vi "Launch.vi"(6 "Only Init (F)":bool, 7 "API Type (Base)":refnum<class "Actor API.lvclass">, 8 "error in (no error)":errorcluster, 11 "Actor in":refnum<class "Actor.lvclass">) -> (0 "error out":errorcluster, 3 "Actor API":refnum<class "Actor API.lvclass">)   [LabVIEW 2022 SP3, in "Artifex.lvlib" / "Actor.lvclass"]
uses:
  Actor.lvclass
  Priority Message Queue/Priority Message Queue.lvclass
  Actor Proxy/Actor API.lvclass
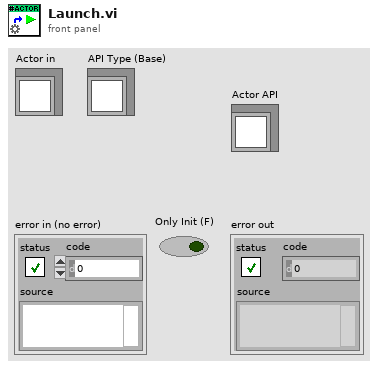
[diagram p1: front panel]
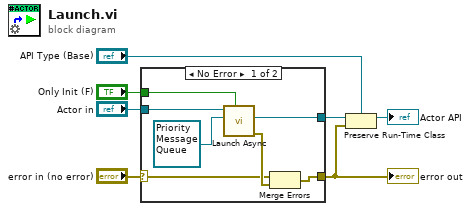
[diagram p0: block diagram]
diagram:
  n1 = case shown="No Error" "error in (no error)" {
    selector: "error in (no error)" -> [w13 w15]
    tunnel: "Actor in" -> [w8 _]
    tunnel: [w12 w15] -> w4
    tunnel: [w10 _] -> w5
    tunnel: "Only Init (F)" -> [w9 _]
    frame No Error {
      n2 = call "Launch Async.vi"("Only Init"=w9, "Caller Queue"=refnum<class "Priority Message Queue.lvclass"> refnum, "Actor in"=w8) -> ("error out"=w14:errorcluster, "Actor API"=w10:refnum<class "Actor API.lvclass">)  [unwired: 7 in]
      n3 = Merge Errors(w13, w14) -> (w12:errorcluster)
    }
    frame Error {
    }
  }
  "error out" <- w4
  n4 = Preserve Run-Time Class(object in=w5, error in=w4, 2:"API Type (Base)") -> (object out=→"Actor API":refnum<class "Actor API.lvclass">)  [unwired: 1 out]
